vi "ExSubNframeCol_new.vi"(8 "error in (no error)":errorcluster, 9 "image handles":u32[](array[numeric]), 10 "Number of Images":u32=1 min=1 step=1, 11 "Handle Cluster 2":T1) -> (0 "error out":errorcluster, 1 "data handles":u32[](array[numeric]), 2 "x/y":dbl, 3 "Handle Cluster":T1)   [LabVIEW 2015]
panel:
  out "image #":i32
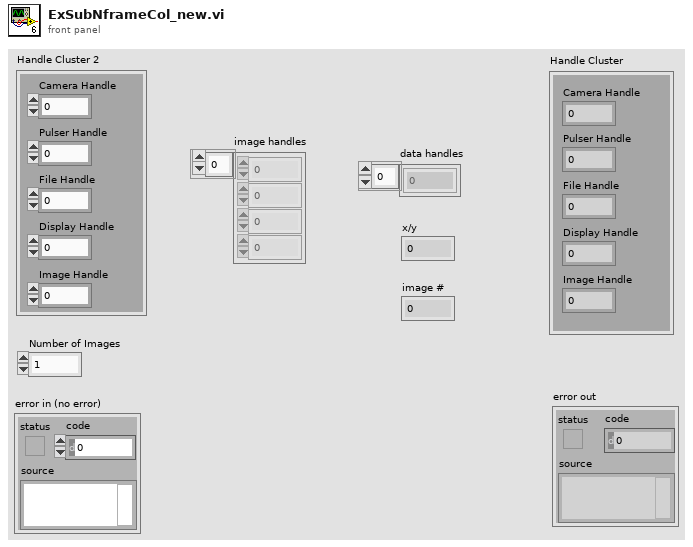
[diagram p1: front panel]
types:
  T1 = cluster{"Camera Handle":u32, "Pulser Handle":u32, "File Handle":u32, "Display Handle":u32, "Image Handle":u32}
  T2 = cluster{"Camera Handle":u32, "Pulser Handle":u32, "File Handle":u32, "Display Handle":u32, "Data Handle":u32}
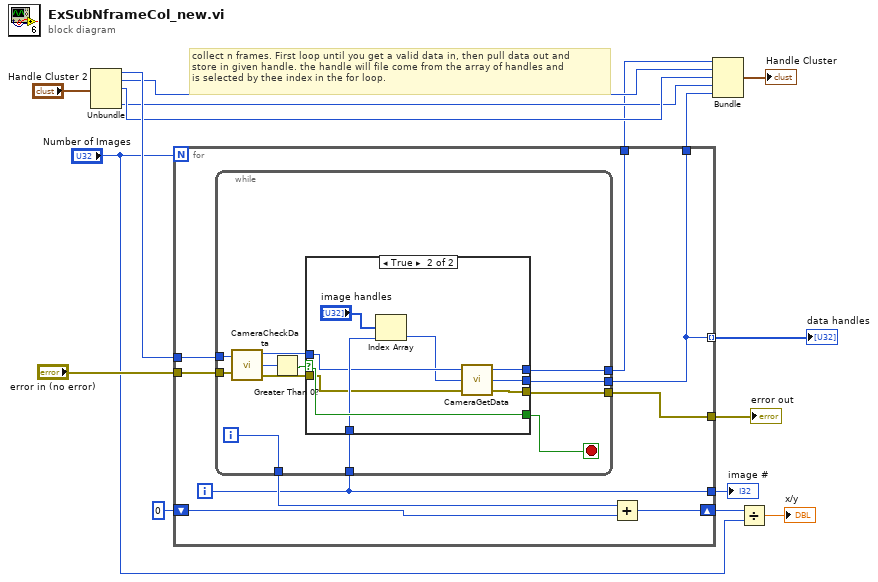
[diagram p0: block diagram]
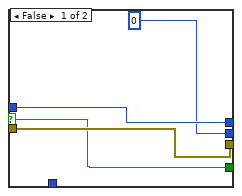
[diagram p2: hidden frame]
diagram:
  # "collect n frames. First loop until you get a valid data in, then pull data out and \nstore in given handle. the handle will file come from the array of handles and\nis selected by thee index in the for loop."
  n1 = Unbundle("Handle Cluster 2") -> ("Camera Handle"=w16:u32, "Pulser Handle"=w13:u32, "File Handle"=w12:u32, "Display Handle"=w11:u32)  [unwired: 1 out]
  n2 = for {
    N: "Number of Images" -> [_]
    tunnel: w16 -> [w25]
    tunnel: "error in (no error)" -> [w24]
    tunnel: [w23] -> w14
    tunnel: [w22] -> w8
    tunnel: [w21] -> w10
    tunnel: [w21] -> w9 mode=indexing
    shift-right: [w20] -> w4
    shift-left: 0 -> [w18]
    tunnel: [w17] -> w1
    i -> [w17]
    n3 = while {
      tunnel: w24 -> [w31]
      tunnel: w25 -> [w32]
      tunnel: [w37] -> w23
      tunnel: w17 -> [w36]
      tunnel: [w35] -> w22
      tunnel: [w34] -> w21
      tunnel: [w27] -> w19
      i -> [w27]
      stop <- w26 stop-if-true
      n4 = call <userlib>:"CameraCheckData.vi"("Camera Handle"=w32, "error in"=w31) -> ("Camera Handle"=w28:u32, "Number Of Frames Available"=w29:i32, "error out"=w30:errorcluster)
      n5 = Greater Than 0?(x=w29) -> (x > 0?=w33:bool)
      n6 = case shown="True" w33 {
        selector: w33 -> [w40 w50]
        tunnel: w28 -> [w39 w47]
        tunnel: w30 -> [w41 w45]
        tunnel: [w40 w50] -> w26
        tunnel: [w41 w42] -> w37
        tunnel: w36 -> [_ w49]
        tunnel: [w39 w44] -> w35
        tunnel: [0 w43] -> w34
        frame False {
        }
        frame True {
          n7 = Index Array(array="image handles", index=w49) -> (element=w46:u32)
          n8 = call <userlib>:"CameraGetData.vi"("error in"=w45, "Data Handle"=w46, "Camera Handle"=w47) -> ("error out"=w42:errorcluster, "Data Handle"=w43:u32, "Camera Handle"=w44:u32)
        }
      }
    }
    n9 = Add(x=w19, y=w18) -> (x+y=w20:i32)
  }
  "error out" <- w14
  "data handles" <- w9
  "image #" <- w1
  n10 = Bundle("Camera Handle"=w8, "Pulser Handle"=w13, "File Handle"=w12, "Display Handle"=w11, "Data Handle"=w10) -> (→"Handle Cluster":T2)  [unwired: 1 in]
  n11 = Divide(x=w4, y="Number of Images") -> (x/y=→"x/y":dbl)
